vi "align_lidar_distance.vi"() -> (3 "PID A":T2(graph)={"Setpoint"=-0.02930742489899981, "output"=0.018032836156553524, "dx/dt"=0.0})   [LabVIEW 2017]
uses:
  <vilib>/myRIO/Instrument Drivers/Utilities/Utilities.lvlib
  <vilib>/myRIO/Express VI/Onboard IO/Encoder/Encoder Express VI.xnode
  <vilib>/myRIO/Instrument Drivers/Onboard IO/Encoder/vis/Read.vi
  <vilib>/myRIO/Instrument Drivers/Onboard IO/Encoder/Encoder.lvlib
  <vilib>/myRIO/Common/Instrument Driver Framework/myRIO v1.0/Encoder/typedefs/Encoder Signal Mode.ctl
  <vilib>/myRIO/Common/Instrument Driver Framework/myRIO v1.0/Encoder/typedefs/Encoder Channels Enum.ctl
  <vilib>/myRIO/Common/Instrument Driver Framework/Utilities/typedefs/Generic FPGA Reference.ctl
  <vilib>/myRIO/Common/Instrument Driver Framework/Utilities/typedefs/myRIO v1.0 Reference.ctl
  <vilib>/myRIO/Common/Instrument Driver Framework/Utilities/typedefs/Hardware Version Enum.ctl
  <vilib>/myRIO/Common/Instrument Driver Framework/Utilities/typedefs/myRIO Generic Hardware Reference.ctl
  <vilib>/myRIO/Instrument Drivers/Onboard IO/Encoder/typedefs/Encoder Reference.ctl
  <vilib>/myRIO/Instrument Drivers/Onboard IO/Encoder/vis/myRIO Encoder Open.xnode
  <vilib>/myRIO/Common/Instrument Driver Framework/Utilities/vis/Is FPGA Ref Available.vi
  <vilib>/myRIO/Common/Instrument Driver Framework/myRIO v1.0/Encoder/vis/myRIO v1.1 Open Encoder.vi
  <vilib>/myRIO/Common/Instrument Driver Framework/myRIO v1.0/Encoder/vis/myRIO v1.0 Configure Encoder.vi
  <vilib>/myRIO/Common/Instrument Driver Framework/myRIO v1.0/Encoder/typedefs/Encoder Configuration v1.0.ctl
  <vilib>/userdefined/High Color/nirio_resource_hc.ctl
  <vilib>/myRIO/Common/Instrument Driver Framework/myRIO v1.0/Encoder/typedefs/Encoder Count Direction Enum.ctl
  <vilib>/addons/control/pid/NI_PID_pid.lvlib
  <vilib>/addons/control/pid/pid.llb/PID (DBL).vi
panel:
  out "Waveform Chart":dbl(graph)
  in  "setpoint":dbl format="%.2f"
  in  "Angle PIDS":T1={"proportional gain (Kc)"=0.05, "integral time (Ti, min)"=0.05, "derivative time (Td, min)"=0.0} {"derivative time (Td, min)" format="%.3f"; "integral time (Ti, min)" format="%.3f"; "proportional gain (Kc)" format="%.3f"}
  in  "stop":bool
  out "OUTPUT B":dbl(slide) scale=-10.0..10.0
  out "OUTPUT A":dbl(slide) scale=-10.0..10.0
  out "PID B":T2(graph)={"Setpoint"=-0.0010415887580554149, "output"=-0.02086159598615355, "dx/dt"=0.0}
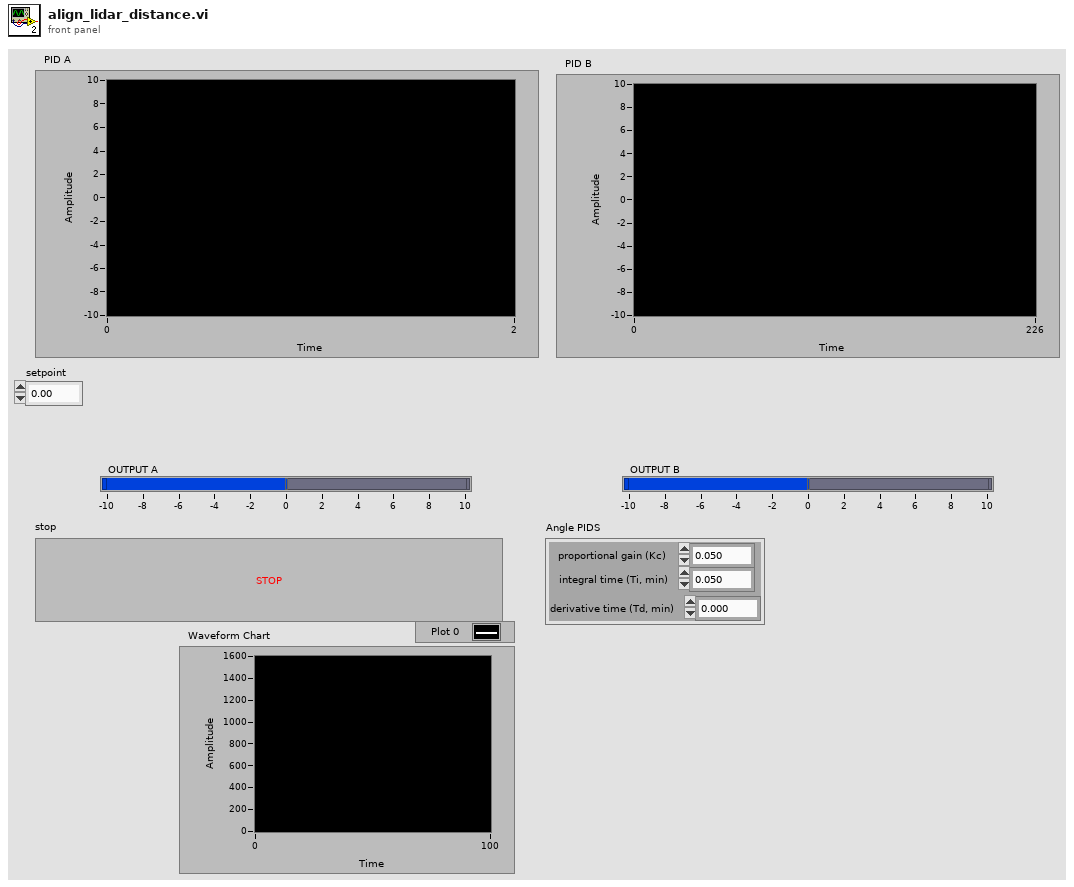
[diagram p1: front panel]
types:
  T1 = cluster{"proportional gain (Kc)":dbl, "integral time (Ti, min)":dbl, "derivative time (Td, min)":dbl}
  T2 = cluster{"Setpoint":dbl, "output":dbl, "dx/dt":dbl}
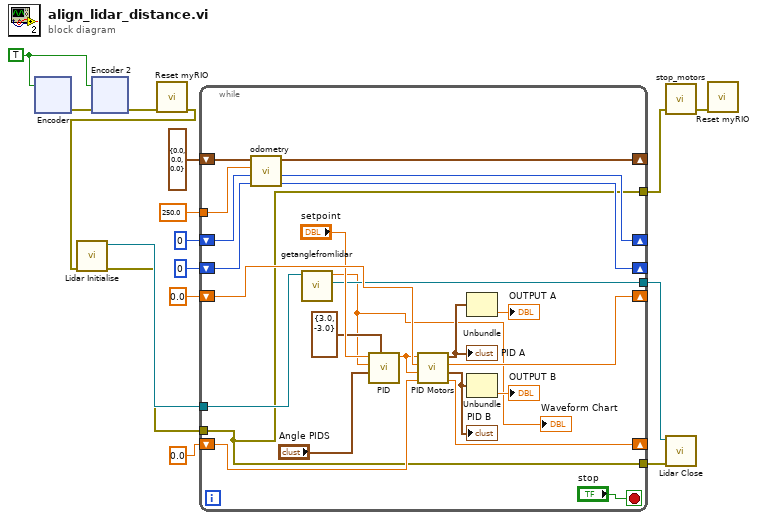
[diagram p0: block diagram]
diagram:
  w14 = TRUE
  n1 = xnode "Encoder"("Reset Counter"=w14) -> ("error out"=w15:errorcluster)  [unwired: 1 in, 3 out]
  n2 = xnode "Encoder 2"("error in (no error)"=w15, "Reset Counter"=w14) -> ("error out"=w16:errorcluster)  [unwired: 3 out]
  n3 = call <vilib>:"Reset myRIO.vi"("error in (no error)"=w16) -> ("error out"=w2:errorcluster)  [unwired: 10 in]
  n4 = call "Lidar Initialise.vi"("error in (no error)"=w2) -> ("error out"=w3:errorcluster, "VISA resource name out"=w5:refnum<visa-resource-name>)  [unwired: 9 in]
  n5 = while {
    shift-right: [w37] -> _
    shift-left: 0.0 ("output A") -> [w38]
    shift-right: [w40] -> _
    shift-left: 0.0 ("output B") -> [w39]
    shift-right: [w30] -> _
    shift-left: 0 ("ENCA OUT") -> [w28]
    shift-right: [w29] -> _
    shift-left: 0 ("ENCB OUT") -> [w27]
    shift-right: [w26] -> _
    shift-left: cluster{dbl, dbl, dbl} {0.0, 0.0, 0.0} ("X, Y, BEARING") -> [w25]
    tunnel: 250.0 ("wheelbase") -> [w24]
    tunnel: w3 -> [w17]
    tunnel: [w17] -> w6
    tunnel: w5 -> [w22]
    tunnel: [w21] -> w4
    tunnel: [w17] -> w1
    stop <- "stop" stop-if-true
    n6 = call "odometry.vi"("ENCB in"=w27, "ENCA in"=w28, "wheelbase"=w24, "Position"=w25) -> ("ENCB OUT"=w29:i32, "ENCA OUT"=w30:i32, "X, Y, BEARING"=w26:cluster{dbl, dbl, dbl})  [unwired: 4 in]
    n7 = call "getanglefromlidar.vi"("VISA resource name"=w22) -> ("VISA resource name out"=w21:refnum<visa-resource-name>, "Distance from Wall"=w18:dbl)  [unwired: 5 in, 4 out]
    "Waveform Chart" <- w18
    n8 = call-poly <vilib>:"PID.vi"("output range"=cluster{"output high":dbl, "output low":dbl} {"output high"=3.0, "output low"=-3.0}, "PID gains"="Angle PIDS", "process variable"=w18, "setpoint"="setpoint") -> ("output"=w20:dbl)  [unwired: 6 in, 1 out]
    n9 = call "PID Motors.vi"("input B"=w39, "Speed B"=w20, "input A"=w38, "Speed A"=w20) -> ("output B"=w40:dbl, "Speed B0"=w35:T2, "output A"=w37:dbl, "Speed A0"=w36:T2)
    "PID B" <- w35
    "PID A" <- w36
    n10 = Unbundle(w36) -> ("dx/dt"=→"OUTPUT A":dbl)  [unwired: 2 out]
    n11 = Unbundle(w35) -> ("dx/dt"=→"OUTPUT B":dbl)  [unwired: 2 out]
  }
  n12 = call "stop_motors.vi"("error in (no error)"=w1) -> ("error out"=w11:errorcluster)  [unwired: 4 in]
  n13 = call "Lidar Close.vi"("error in (no error)"=w6, "VISA resource name"=w4) -> ()  [unwired: 9 in, 1 out]
  n14 = call <vilib>:"Reset myRIO.vi"("error in (no error)"=w11) -> ()  [unwired: 10 in, 1 out]
